vi "Convert Data.vi"(6 "Data Type (1 : Int)":i32(ring)=1 items=["NULL", "INT", "FLOAT"], 8 "error in (no error)":errorcluster, 9 "Decimal Position (0)":i32 min=0 max=4 step=1, 10 "Integer Data (0)":i32, 11 "VISA resource name":refnum<visa-resource-name>) -> (0 "error out":errorcluster, 2 "Float Data":dbl format="%#.4f", 3 "VISA resource name out":refnum<visa-resource-name>)   [LabVIEW 2020, in "Yokogawa GX Series.lvlib"]
doc: "This VI converts Integer Data that is a part of Measurement Block Data (Measurement Binary Data) and Decimal Position to a floating-point number."
uses:
  <instrlib>/Yokogawa GX Series/Yokogawa GX Series.lvlib
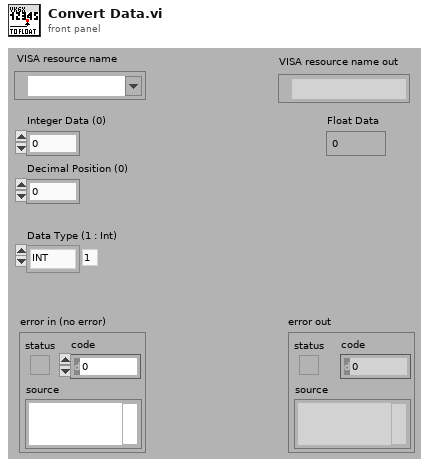
[diagram p1: front panel]
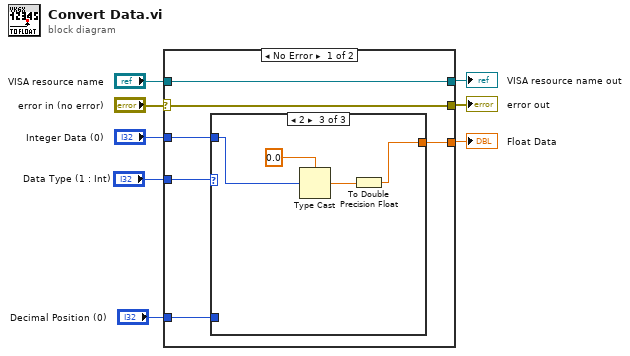
[diagram p0: block diagram]
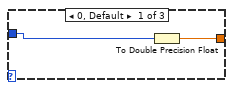
[diagram p2: hidden frame]
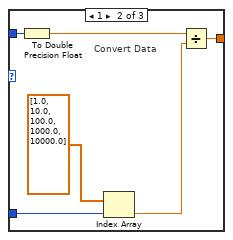
[diagram p3: hidden frame]
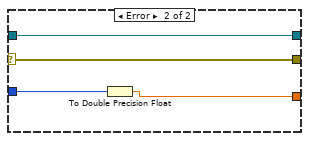
[diagram p4: hidden frame]
diagram:
  n1 = case shown="No Error" "error in (no error)" {
    selector: "error in (no error)" -> [w10 w27]
    tunnel: "Integer Data (0)" -> [w14 w30]
    tunnel: [w13 w29] -> w7
    tunnel: "Decimal Position (0)" -> [w12 _]
    tunnel: "VISA resource name" -> [w11 w28]
    tunnel: [w11 w28] -> w4
    tunnel: [w10 w27] -> w2
    tunnel: "Data Type (1 : Int)" -> [w9 _]
    frame No Error {
      n2 = case shown="2" w9 {
        tunnel: w14 -> [w16 w22 w26]
        tunnel: [w15 w21 w23] -> w13
        tunnel: w12 -> [_ w20 _]
        frame 0, Default {
          n3 = To Double Precision Float(number=w16) -> (double precision float=w15:dbl)
        }
        frame 1 {
          # "Convert Data"
          n4 = To Double Precision Float(number=w22) -> (double precision float=w18:dbl)
          n5 = Index Array(array=dbl[] [1.0, 10.0, 100.0, 1000.0, 10000.0], index=w20) -> (element=w19:dbl)
          n6 = Divide(x=w18, y=w19) -> (x/y=w21:dbl)
        }
        frame 2 {
          n7 = Type Cast(type=sgl 0.0, x=w26) -> (*(type *) &x=w24:sgl)
          n8 = To Double Precision Float(number=w24) -> (double precision float=w23:dbl)
        }
      }
    }
    frame Error {
      n9 = To Double Precision Float(number=w30) -> (double precision float=w29:dbl)
    }
  }
  "Float Data" <- w7
  "VISA resource name out" <- w4
  "error out" <- w2
